vi "ON-1CH.vi"(1 "CH(0-63)":i32 min=0 max=63, 2 "lines":tag="Dev2/port0/line0:7") -> (0 "Status(U8)":u8)   [LabVIEW 2020]
uses:
  <vilib>/DAQmx/write.llb/DAQmx Write (Digital U8 1Chan 1Samp).vi
  <vilib>/DAQmx/create/channels.llb/DAQmx Create Channel (DO-Digital Output).vi
  <vilib>/DAQmx/miscellaneous.llb/DAQmx Fill In Error Info.vi
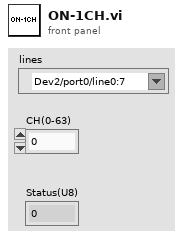
[diagram p1: front panel]
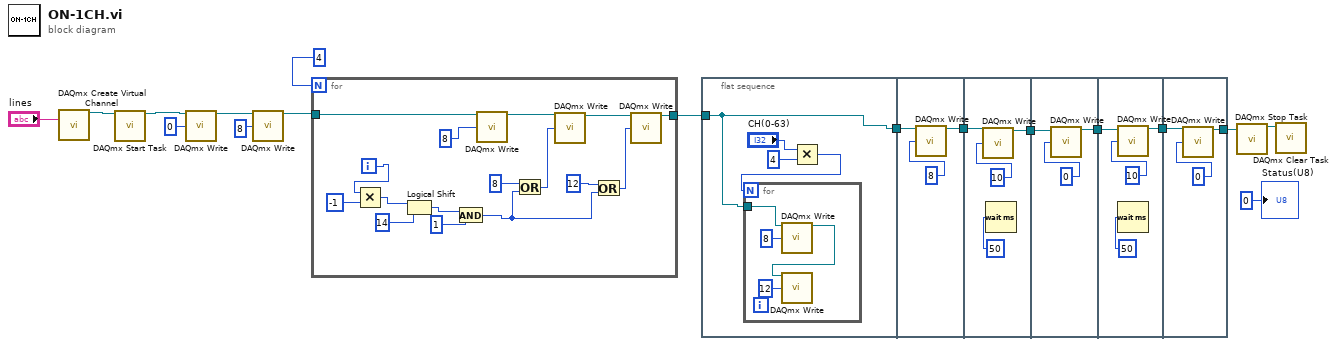
[diagram p0: block diagram]
diagram:
  n1 = call-poly <vilib>:"DAQmx Create Virtual Channel.vi"("lines"="lines") -> ("task out"=w17:refnum<k21>)  [unwired: 13 in, 1 out]
  n2 = call <vilib>:"DAQmx Start Task.vi"("task/channels in"=w17) -> ("task out"=w11:refnum<k21>)  [unwired: 13 in, 1 out]
  n3 = call-poly <vilib>:"DAQmx Write.vi"("task/channels in"=w11, "data"=u8 0) -> ("task out"=w10:refnum<k21>)  [unwired: 11 in, 2 out]
  n4 = call-poly <vilib>:"DAQmx Write.vi"("task/channels in"=w10, "data"=u8 8) -> ("task out"=w13:refnum<k21>)  [unwired: 11 in, 2 out]
  n5 = for {
    N: 4 -> [_]
    tunnel: w13 -> [w22]
    tunnel: [w19] -> w2
    i -> [w31]
    n6 = Multiply(x=w31, y=-1) -> (x*y=w29:i32)
    n7 = Logical Shift(y=w29, x=u8 14) -> (x << y=w33:u8)
    n8 = And(x=w33, y=u32 1) -> (x .and. y?=w25:u32)
    n9 = call-poly <vilib>:"DAQmx Write.vi"("task/channels in"=w22, "data"=u32 8 ("x")) -> ("task out"=w21:refnum<k21>)  [unwired: 11 in, 2 out]
    n10 = Or(x=u32 8, y=w25) -> (x .or. y?=w26:u32)
    n11 = call-poly <vilib>:"DAQmx Write.vi"("task/channels in"=w21, "data"=w26) -> ("task out"=w20:refnum<k21>)  [unwired: 11 in, 2 out]
    n12 = Or(x=u32 12, y=w25) -> (x .or. y?=w23:u32)
    n13 = call-poly <vilib>:"DAQmx Write.vi"("task/channels in"=w20, "data"=w23) -> ("task out"=w19:refnum<k21>)  [unwired: 11 in, 2 out]
  }
  n14 = flat-sequence {
    tunnel: [w34] -> w3
    tunnel: w2 -> [w34]
    tunnel: [w42] -> w8
    tunnel: w3 -> [w43]
    tunnel: w8 -> [w46]
    tunnel: [w45] -> w7
    tunnel: w7 -> [w50]
    tunnel: [w49] -> w6
    tunnel: w6 -> [w53]
    tunnel: [w52] -> w5
    tunnel: w5 -> [w57]
    tunnel: [w56] -> w4
    frame #0 {
      n15 = Multiply(x="CH(0-63)", y=4) -> (x*y=w37:i32)
      n16 = for {
        N: w37 -> [_]
        tunnel: w34 -> [w39]
        n17 = call-poly <vilib>:"DAQmx Write.vi"("task/channels in"=w39, "data"=u8 8) -> ("task out"=w38:refnum<k21>)  [unwired: 11 in, 2 out]
        n18 = call-poly <vilib>:"DAQmx Write.vi"("task/channels in"=w38, "data"=u8 12) -> ()  [unwired: 11 in, 3 out]
      }
    }
    frame #1 {
      n19 = call-poly <vilib>:"DAQmx Write.vi"("task/channels in"=w43, "data"=u8 8) -> ("task out"=w42:refnum<k21>)  [unwired: 11 in, 2 out]
    }
    frame #2 {
      n20 = call-poly <vilib>:"DAQmx Write.vi"("task/channels in"=w46, "data"=u8 10) -> ("task out"=w45:refnum<k21>)  [unwired: 11 in, 2 out]
      n21 = Wait (ms)(milliseconds to wait=u32 50) -> ()  [unwired: 1 out]
    }
    frame #3 {
      n22 = call-poly <vilib>:"DAQmx Write.vi"("task/channels in"=w50, "data"=u8 0) -> ("task out"=w49:refnum<k21>)  [unwired: 11 in, 2 out]
    }
    frame #4 {
      n23 = call-poly <vilib>:"DAQmx Write.vi"("task/channels in"=w53, "data"=u8 10) -> ("task out"=w52:refnum<k21>)  [unwired: 11 in, 2 out]
      n24 = Wait (ms)(milliseconds to wait=u32 50) -> ()  [unwired: 1 out]
    }
    frame #5 {
      n25 = call-poly <vilib>:"DAQmx Write.vi"("task/channels in"=w57, "data"=u8 0) -> ("task out"=w56:refnum<k21>)  [unwired: 11 in, 2 out]
    }
  }
  n26 = call <vilib>:"DAQmx Stop Task.vi"("task/channels in"=w4) -> ("task out"=w16:refnum<k21>)  [unwired: 13 in, 1 out]
  n27 = call <vilib>:"DAQmx Clear Task.vi"("task in"=w16) -> ()  [unwired: 14 in, 1 out]
  "Status(U8)" <- u8 0
